vi "FFTData To Waveform.vi"(11 "FFT":cluster{"f0":dbl, "df":dbl, "real part":dbl[]}[](array[cluster])) -> (3 "Waveform Data":waveform(dbl)[](array[waveform]))   [LabVIEW 2017]
doc: "Converts FFT data into waveforms, mapping f0 to t0, df to dt and the real part to Y."
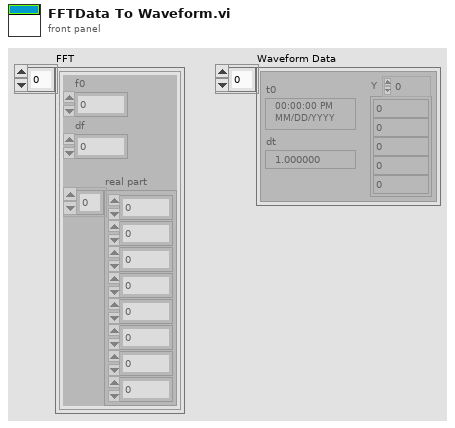
[diagram p1: front panel]
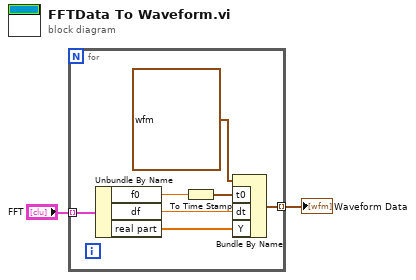
[diagram p0: block diagram]
diagram:
  n1 = for {
    tunnel: "FFT" -> [w8] mode=indexing
    tunnel: [w3] -> w1 mode=indexing
    n2 = Unbundle By Name(w8) -> ("f0"=w7:dbl, "df"=w6:dbl, "real part"=w5:dbl[])
    n3 = To Time Stamp(1:w7) -> (0:w4:timestamp)
    n4 = Bundle By Name(cluster=waveform(dbl) {"t0"=timestamp(0 s since 1904-01-01), "dt"=1.0, "Y"=[]} ("Waveform"), "t0"=w4, "dt"=w6, "Y"=w5) -> (w3:waveform(dbl))
  }
  "Waveform Data" <- w1
